vi "Sort Array Optimised.vi"(1 "Array In":dbl[](array[numeric])) -> (0 "Sorted Array out":dbl[](array[numeric]))   [LabVIEW 2015]
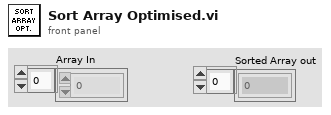
[diagram p1: front panel]
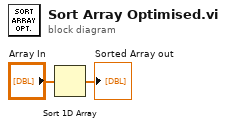
[diagram p0: block diagram]
diagram:
  n1 = Sort 1D Array(array="Array In") -> (sorted array=→"Sorted Array out":dbl[])
